vi "Launch Setting.vi"(8 "error in (no error)":errorcluster, 11 "[V] Main UI in":refnum<class "[V] Main UI.lvclass">) -> (0 "error out":errorcluster, 3 "[V] Main UI out":refnum<class "[V] Main UI.lvclass">)   [LabVIEW 2020, in "[V] Main UI.lvlib" / "[V] Main UI.lvclass"]
uses:
  [V] Main UI.lvclass
  Setting View/Setting View/Setting View.lvclass
  C:/Program Files (x86)/National Instruments/LabVIEW 2020/vi.lib/ActorFramework/Actor/Actor.lvclass
  <vilib>/ActorFramework/Message Enqueuer/Message Enqueuer.lvclass/Message Enqueuer.ctl
  <vilib>/ActorFramework/Message Enqueuer/Enqueue.vi
  Depden On/Abstruct View/Abstruct View Messages/Show Front Msg/Show Front Msg.lvclass
  C:/Program Files (x86)/National Instruments/LabVIEW 2020/vi.lib/ActorFramework/Message/Message.lvclass
  <vilib>/ActorFramework/Message Priority Queue/Priority Enqueue.vi
  [V] Main UI.lvclass/[V] Main UI.ctl
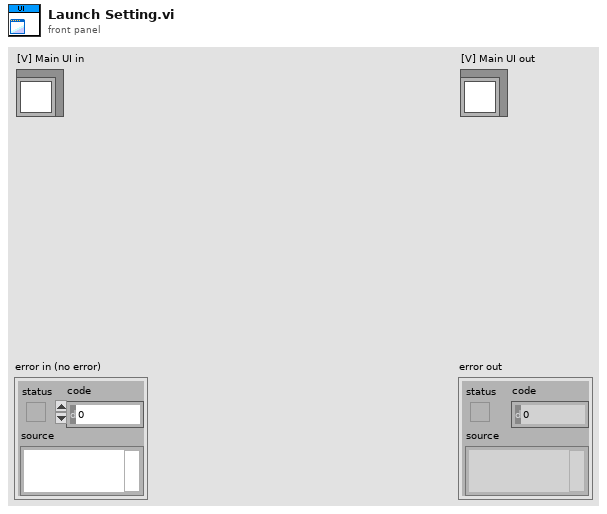
[diagram p1: front panel]
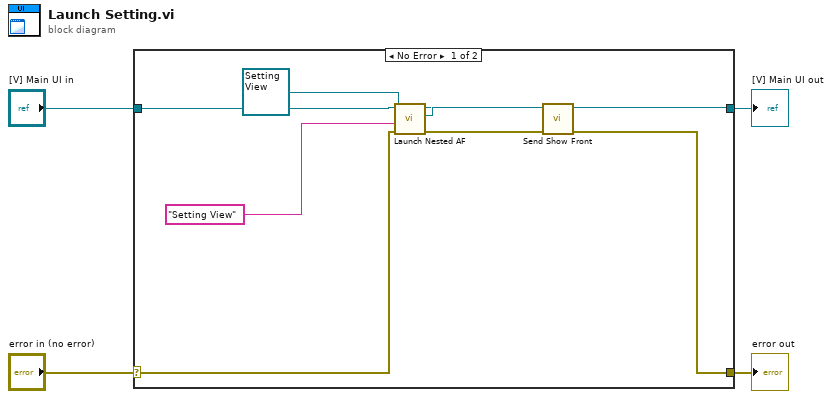
[diagram p0: block diagram]
diagram:
  n1 = case shown="No Error" "error in (no error)" {
    selector: "error in (no error)" -> [w7 w14]
    tunnel: [w5 w14] -> w3
    tunnel: [w8 w13] -> w1
    tunnel: "[V] Main UI in" -> [w12 w13]
    frame No Error {
      n2 = call "Launch Nested AF.vi"("error in (no error)"=w7, "name"="Setting View", "Nested Actor"=refnum<class "Setting View.lvclass"> refnum ("[V]Setting View.lvlib:Setting View.lvclass"), "[V] Main UI in"=w12) -> ("error out"=w6:errorcluster, "Enqueuer"=w11:refnum<class "Message Enqueuer.lvclass">, "[V] Main UI out"=w8:refnum<class "[V] Main UI.lvclass">)  [unwired: 5 in]
      n3 = call "Send Show Front.vi"("error in (no error)"=w6, "Message Enqueuer"=w11) -> ("error out"=w5:errorcluster)  [unwired: 8 in, 1 out]
    }
    frame Error {
    }
  }
  "error out" <- w3
  "[V] Main UI out" <- w1
